vi "Password_Prompt.vi"(0 "Enable":bool=TRUE, 5 "error in (no error)":errorcluster) -> (17 "Password":string, 18 "OK":bool, 19 "error out":errorcluster)   [LabVIEW 2020]
doc: "Displays a standard dialog box that prompts users to enter information, such as a user name and password.\n--------------------\n\nThis Express VI is configured as follows:\n\nMessage to Display to the User:Insert Password\nThe inputs are: \nText Entry Box: Password"
uses:
  <vilib>/Utility/inputDevices.llb/keyboardAcquire.vi
panel:
  in  "Enter password:":string caption="Password"
  out "String":string="Insert Password"
  in  "Cancel":bool
  in  "OK2":bool
  in  "OK1":bool
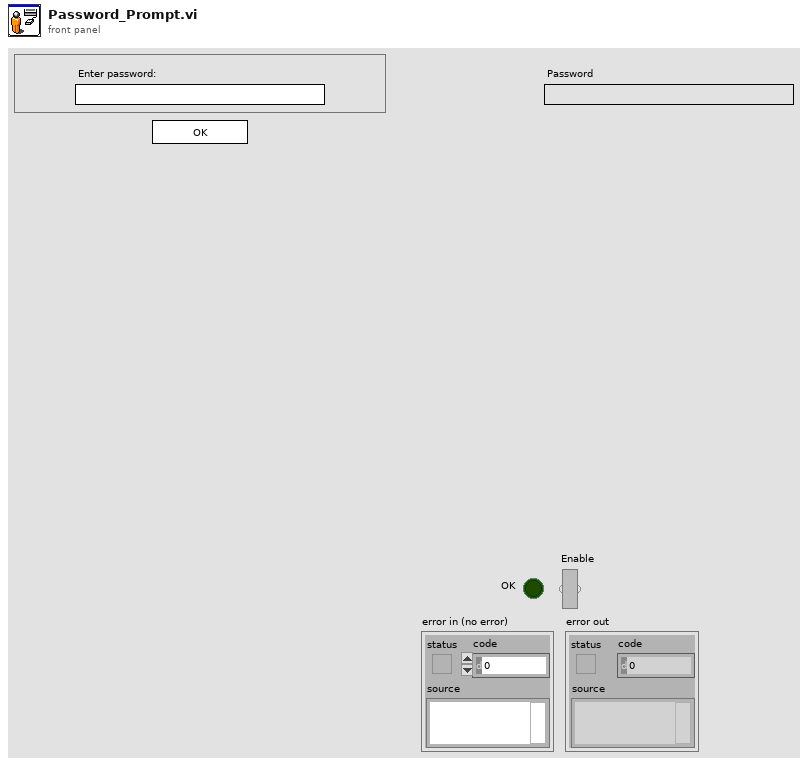
[diagram p1: front panel]
types:
  T1 = cluster{"Input Name":string, "Input Data Type":i32}[]
  T2 = enum16{"0", "1", "2", "3", "4", "5", "6", "7", "8", "9", "A", "B", "C", "D", "E", "F", "G", "H", "I", "J", "K", "L", "M", "N", "O", "P", "Q", "R", "S", "T", "U", "V", "W", "X", "Y", "Z", "F1", "F2", "F3", "F4", "F5", "F6", "F7", "F8", "F9", "F10", "F11", "F12", "F13", "F14", "F15", "ADD", "BACK", "BACKSLASH", "CAPITAL", "COMMA", "DECIMAL", "DELETE", "DIVIDE", "DOWN", "END", "EQUALS", "ESCAPE", "GRAVE (`)", "HOME", "INSERT", "LBRACKET", "LCONTROL", "LEFT", "L ALT", "LSHIFT", "LWIN", "MINUS", "MULTIPLY", "NEXT", "NUMLOCK", "NUMPAD_0", "NUMPAD_1", "NUMPAD_2", "NUMPAD_3", "NUMPAD_4", "NUMPAD_5", "NUMPAD_6", "NUMPAD_7", "NUMPAD_8", "NUMPAD_9", "PAUSE", "PERIOD", "PRIOR (PG UP)", "RBRACKET", "RCONTROL", "RETURN", "RIGHT", "R ALT", "RSHIFT", "RWIN", "SCROLL", "SEMICOLON", "SLASH", "SPACE", "SUBTRACT", "TAB", "UP", "ENTER (num pad)", "' (quote)"}
  T3 = enum16{"0", "1", "2", "3", "4", "5", "6", "7", "8", "9", "A", "B", "C", "D", "E", "F", "G", "H", "I", "J", "K", "L", "M", "N", "O", "P", "Q", "R", "S", "T", "U", "V", "W", "X", "Y", "Z", "F1", "F2", "F3", "F4", "F5", "F6", "F7", "F8", "F9", "F10", "F11", "F12", "F13", "F14", "F15", "ADD", "BACK", "BACKSLASH", "CAPITAL", "COMMA", "DECIMAL", "DELETE", "DIVIDE", "DOWN", "END", "EQUALS", "ESCAPE", "GRAVE (`)", "HOME", "INSERT", "LBRACKET", "LCONTROL", "LEFT", "L ALT", "LSHIFT", "LWIN", "MINUS", "MULTIPLY", "NEXT", "NUMLOCK", "NUMPAD_0", "NUMPAD_1", "NUMPAD_2", "NUMPAD_3", "NUMPAD_4", "NUMPAD_5", "NUMPAD_6", "NUMPAD_7", "NUMPAD_8", "NUMPAD_9", "PAUSE", "PERIOD", "PRIOR (PG UP)", "RBRACKET", "RCONTROL", "RETURN", "RIGHT", "R ALT", "RSHIFT", "RWIN", "SCROLL", "SEMICOLON", "SLASH", "SPACE", "SUBTRACT", "TAB", "UP", "ENTER (num pad)", "' (quote)"}[]
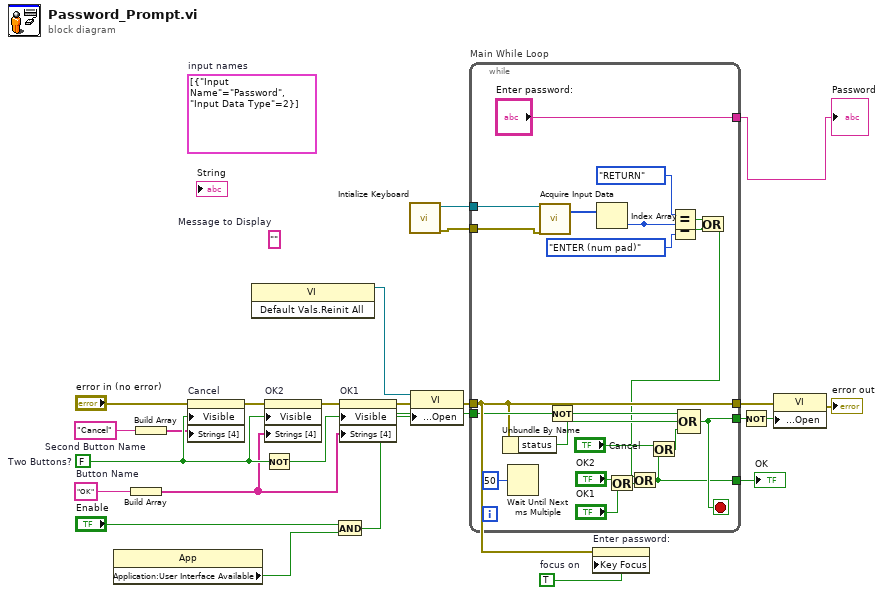
[diagram p0: block diagram]
diagram:
  w4 = TRUE  # focus on
  (unwired) T1 [{"Input Name"="Password", "Input Data Type"=2}]  # input names
  w16 = "Cancel"  # Second Button Name
  w14 = "OK"  # Button Name
  (unwired) ""  # Message to Display
  w24 = FALSE  # Two Buttons?
  n1 = property class="App"() -> ("Application:User Interface Available"=w6:bool)  [unwired: 2 in, 2 out]
  n2 = Build Array(w14) -> (w15:string[])
  n3 = Build Array(w16) -> (w17:string[])
  n4 = property on="Cancel" class="Bool"(error in="error in (no error)", "Visible"=w24, "Strings [4]"=w17) -> (error out=w21:errorcluster)  [unwired: 1 in, 1 out]
  n5 = invoke class="VI" method="Default Vals.Reinit All"() -> (reference out=w5:refnum<vi>)  [unwired: 3 in, 2 out]
  n6 = Not(x=w24) -> (.not. x?=w22:bool)
  n7 = property on="OK2" class="Bool"(error in=w21, "Visible"=w24, "Strings [4]"=w15) -> (error out=w20:errorcluster)  [unwired: 1 in, 1 out]
  n8 = And(x="Enable", y=w6) -> (x .and. y?=w7:bool)
  n9 = property on="OK1" class="Bool"(error in=w20, "Visible"=w22, "Strings [4]"=w15) -> (error out=w13:errorcluster)  [unwired: 1 in, 1 out]
  n10 = call <vilib>:"Intialize Keyboard.vi"() -> ("error out"=w2:errorcluster, "device ID"=w3:refnum<k1>)  [unwired: 10 in]
  n11 = property class="VI"(reference=w5, error in=w13, "Front Panel Window:Open"=w7) -> (error out=w12:errorcluster)  [unwired: 1 out]
  n12 = while "Main While Loop" {
    tunnel: [w34] -> w23
    tunnel: w7 -> [w42]
    tunnel: [w40] -> w18
    tunnel: w12 -> [w39]
    tunnel: [w39] -> w10
    tunnel: ["Enter password:"] -> w1
    tunnel: w3 -> [w33]
    tunnel: w2 -> [w32]
    stop <- w40 stop-if-true
    n13 = Unbundle By Name(w39) -> ("status"=w37:bool)
    n14 = Wait Until Next ms Multiple(millisecond multiple=u32 50) -> ()  [unwired: 1 out]
    n15 = call-poly <vilib>:"Acquire Input Data.vi"("device ID"=w33, "error in (no error)"=w32) -> ("keys pressed"=w31:T3)  [unwired: 15 in, 2 out]
    n16 = Not(x=w42) -> (.not. x?=w41:bool)
    n17 = Index Array(array=w31) -> (element=w28:T2)  [unwired: 1 in]
    n18 = Or(x="OK2", y="OK1") -> (x .or. y?=w35:bool)
    n19 = Equal?(x=T2."RETURN" ("element"), y=w28) -> (x = y?=w27:bool)
    n20 = Equal?(x=w28, y=T2."ENTER (num pad)" ("element")) -> (x = y?=w26:bool)
    n21 = Or(x=w27, y=w26) -> (x .or. y?=w25:bool)
    n22 = Or(x=w25, y=w35) -> (x .or. y?=w34:bool)
    n23 = Or(x="Cancel", y=w34) -> (x .or. y?=w38:bool)
    n24 = Compound Arithmetic op=OR(w41, w37, w38) -> (w40:bool)
  }
  "OK" <- w23
  "Password" <- w1
  n25 = property on="Enter password:" class="Str"(error in=w12, "Key Focus"=w4) -> ()  [unwired: 1 in, 2 out]
  n26 = Not(x=w18) -> (.not. x?=w19:bool)
  n27 = property class="VI"(error in=w10, "Front Panel Window:Open"=w19) -> (error out=→"error out":errorcluster)  [unwired: 1 in, 1 out]
